vi "PBPCIcard_load.vi"(0 "PulseBlaster\nVLIW Array":T1(array[cluster])=[{"Output Bits"=16777215, "Data Field"=0, "OP Code"=0, "Delay Count"=20}, {"Output Bits"=0, "Data Field"=0, "OP Code"=3, "Delay Count"=20}, {"Output Bits"=0, "Data Field"=0, "OP Code"=6, "Delay Count"=60}] {"OP Code" format="%.0x"; "Output Bits" format="%.0x"}, 1 "Bytes/Word":u8=10, 2 "Memory":bool, 3 "error in (no error)":errorcluster, 4 "Base Address":u32 format="%.0x") -> (7 "error out":errorcluster)   [LabVIEW 2013]
doc: "PBcard_load: \nThis vi \n1) resets the PB, (consists of 4 steps)\n2) writes an array of VLIW's (very long instruction word) to the PB memory\n3) sends \"program finished\".\nAfter completion, a \"start\" command to the PB will make it run the programmed sequence. \n\nThe VLIW is implemented as a cluster of four integers (24bit, 20bit, 4bit, 32bit).\n\nNOTE: NO ERROR CHECKING IS PERFORMED. Error checking is supposedly taken care of before the VLIW array image is made, for example by Add_VLIW, which writes a PulseBlaster command to an array in memory. An"
uses:
  pbcomm8.vi
  pbcomm16.vi
  pbcomm32.vi
panel:
  # "External"
  # "Internal"
  # "(24 bits)"
  # "(20 bits)"
  # "(4 bits)"
  # "(32 bits)"
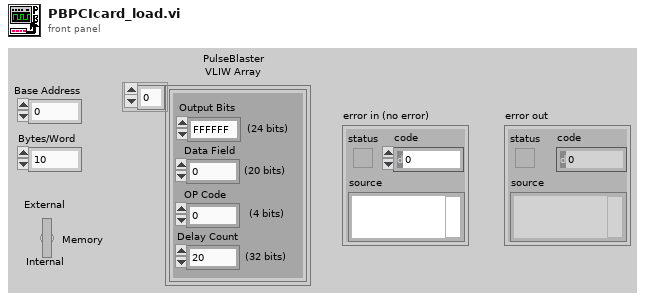
[diagram p1: front panel]
types:
  T1 = cluster{"Output Bits":u32, "Data Field":u32, "OP Code":u8, "Delay Count":u32}[]
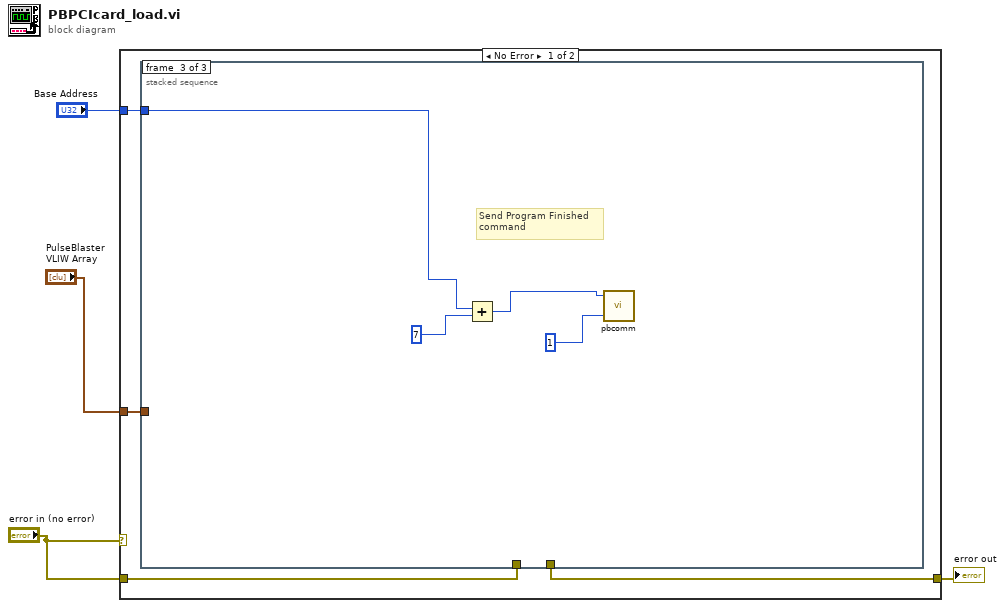
[diagram p0: block diagram]
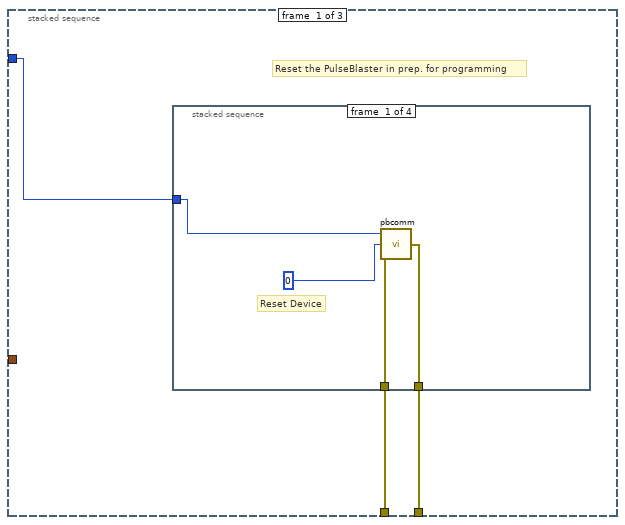
[diagram p2: hidden frame]
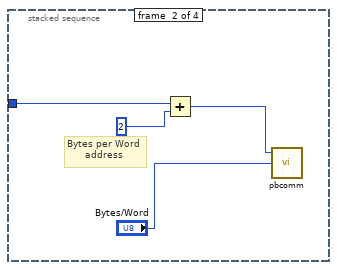
[diagram p3: hidden frame]
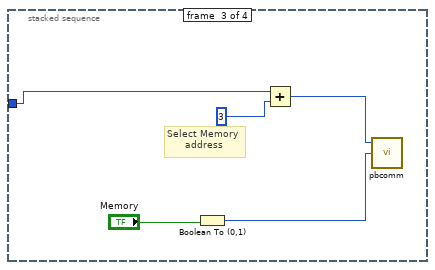
[diagram p4: hidden frame]
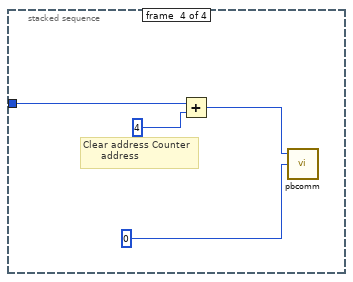
[diagram p5: hidden frame]
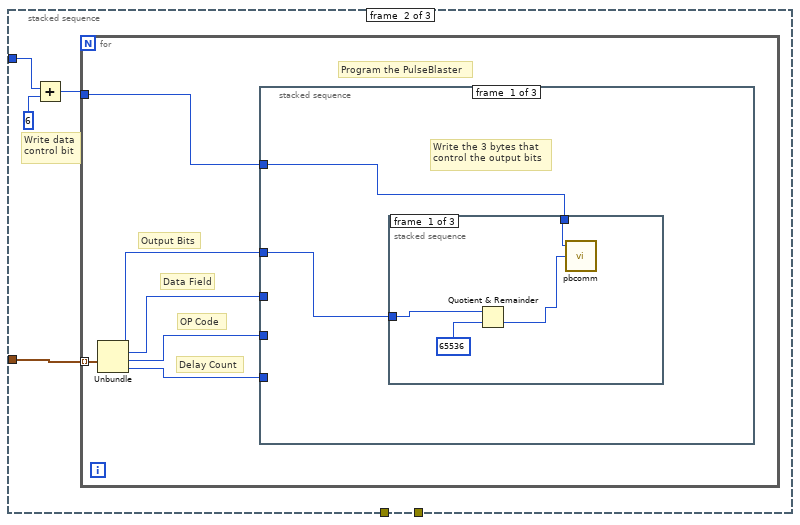
[diagram p6: hidden frame]
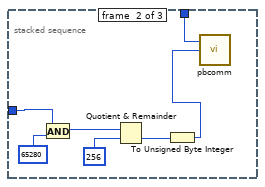
[diagram p7: hidden frame]
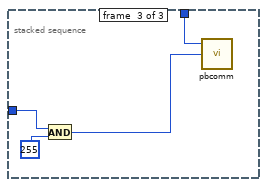
[diagram p8: hidden frame]
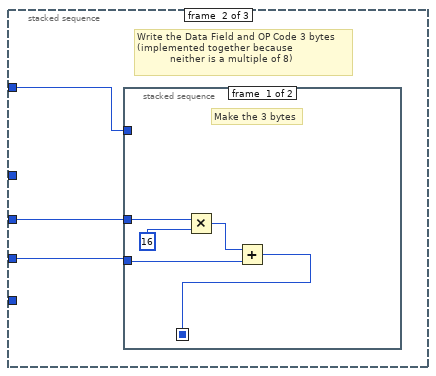
[diagram p9: hidden frame]
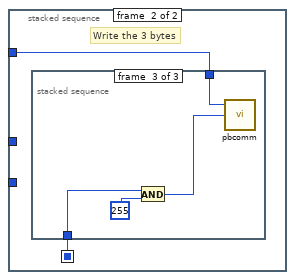
[diagram p10: hidden frame]
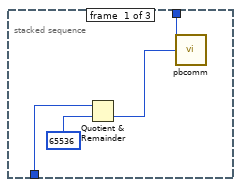
[diagram p11: hidden frame]
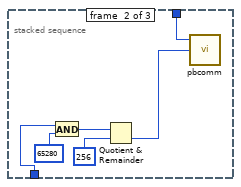
[diagram p12: hidden frame]
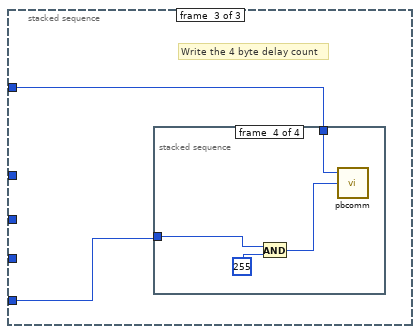
[diagram p13: hidden frame]
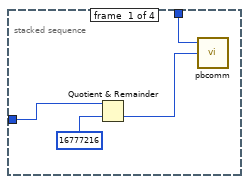
[diagram p14: hidden frame]
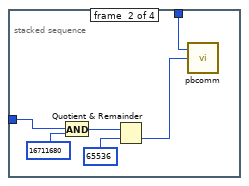
[diagram p15: hidden frame]
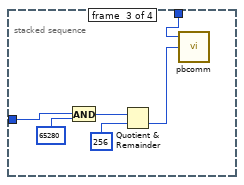
[diagram p16: hidden frame]
diagram:
  n1 = case shown="No Error" "error in (no error)" {
    tunnel: "PulseBlaster\nVLIW Array" -> [w8 _]
    tunnel: "Base Address" -> [w7 _]
    tunnel: "error in (no error)" -> [w6 w106]
    tunnel: [w5 w106] -> w1
    frame No Error {
      n2 = stacked-sequence {
        tunnel: w8 -> [_ w29 _]
        tunnel: w7 -> [w11 w31 w102]
        tunnel: w6 -> [w10 _ _]
        tunnel: [w9 _ _] -> w5
        frame #0 {
          # "Reset the PulseBlaster in prep. for programming"
          n3 = stacked-sequence {
            tunnel: w11 -> [w15 w19 w21 w25]
            tunnel: w10 -> [w13 _ _ _]
            tunnel: [w12 _ _ _] -> w9
            frame #0 {
              # "Reset Device"
              n4 = call-poly "pbcomm.vi"("error in"=w13, "write value"=u8 0, "address"=w15) -> ("error out"=w12:errorcluster)
            }
            frame #1 {
              # "Bytes per Word\n      address"
              n5 = Add(x=w19, y=u8 2) -> (x+y=w17:u32)
              n6 = call-poly "pbcomm.vi"("write value"="Bytes/Word", "address"=w17) -> ()  [unwired: 1 in, 1 out]
            }
            frame #2 {
              # "Select Memory\n      address"
              n7 = Boolean To (0,1)(Boolean="Memory") -> (0, 1=w20:i16)
              n8 = Add(x=w21, y=u8 3) -> (x+y=w23:u32)
              n9 = call-poly "pbcomm.vi"("write value"=w20, "address"=w23) -> ()  [unwired: 1 in, 1 out]
            }
            frame #3 {
              # "Clear address Counter\n      address"
              n10 = Add(x=w25, y=u8 4) -> (x+y=w27:u32)
              n11 = call-poly "pbcomm.vi"("write value"=u8 0, "address"=w27) -> ()  [unwired: 1 in, 1 out]
            }
          }
        }
        frame #1 {
          # "Write data\ncontrol bit"
          n12 = Add(x=w31, y=6) -> (x+y=w30:u32)
          n13 = for {
            tunnel: w30 -> [w38]
            tunnel: w29 -> [w33] mode=indexing
            # "Program the PulseBlaster"
            # "Delay Count"
            # "OP Code"
            # "Data Field"
            # "Output Bits"
            n14 = Unbundle(w33) -> ("Output Bits"=w37:u32, "Data Field"=w36:u32, "OP Code"=w35:u8, "Delay Count"=w34:u32)
            n15 = stacked-sequence {
              tunnel: w37 -> [w40 _ _]
              tunnel: w36 -> [_ w58 _]
              tunnel: w35 -> [_ w57 _]
              tunnel: w38 -> [w39 w56 w80]
              tunnel: w34 -> [_ _ w81]
              frame #0 {
                # "Write the 3 bytes that \ncontrol the output bits"
                n16 = stacked-sequence {
                  tunnel: w40 -> [w43 w49 w54]
                  tunnel: w39 -> [w42 w47 w52]
                  frame #0 {
                    n17 = Quotient & Remainder(x=w43, y=u32 65536) -> (floor(x/y)=w41:u32)  [unwired: 1 out]
                    n18 = call-poly "pbcomm.vi"("write value"=w41, "address"=w42) -> ()  [unwired: 1 in, 1 out]
                  }
                  frame #1 {
                    n19 = And(x=w49, y=u32 65280) -> (x .and. y?=w48:u32)
                    n20 = Quotient & Remainder(x=w48, y=u32 256) -> (floor(x/y)=w46:u32)  [unwired: 1 out]
                    n21 = To Unsigned Byte Integer(number=w46) -> (unsigned 8bit integer=w45:u8)
                    n22 = call-poly "pbcomm.vi"("write value"=w45, "address"=w47) -> ()  [unwired: 1 in, 1 out]
                  }
                  frame #2 {
                    n23 = And(x=w54, y=u32 255) -> (x .and. y?=w53:u32)
                    n24 = call-poly "pbcomm.vi"("write value"=w53, "address"=w52) -> ()  [unwired: 1 in, 1 out]
                  }
                }
              }
              frame #1 {
                # "Write the Data Field and OP Code 3 bytes\n(implemented together because \n           neither is a multiple of 8)"
                n25 = stacked-sequence {
                  seq-local: [w59 _] -> [_ w65]
                  tunnel: w58 -> [w61 _]
                  tunnel: w57 -> [w62 _]
                  tunnel: w56 -> [_ w64]
                  frame #0 {
                    # "Make the 3 bytes"
                    n26 = Multiply(x=w61, y=u32 16) -> (x*y=w60:u32)
                    n27 = Add(x=w60, y=w62) -> (x+y=w59:u32)
                  }
                  frame #1 {
                    # "Write the 3 bytes"
                    n28 = stacked-sequence {
                      tunnel: w65 -> [w67 w71 w77]
                      tunnel: w64 -> [w66 w70 w76]
                      frame #0 {
                        n29 = Quotient & Remainder(x=w67, y=u32 65536) -> (floor(x/y)=w68:u32)  [unwired: 1 out]
                        n30 = call-poly "pbcomm.vi"("write value"=w68, "address"=w66) -> ()  [unwired: 1 in, 1 out]
                      }
                      frame #1 {
                        n31 = And(x=w71, y=u32 65280) -> (x .and. y?=w73:u32)
                        n32 = Quotient & Remainder(x=w73, y=u32 256) -> (floor(x/y)=w72:u32)  [unwired: 1 out]
                        n33 = call-poly "pbcomm.vi"("write value"=w72, "address"=w70) -> ()  [unwired: 1 in, 1 out]
                      }
                      frame #2 {
                        n34 = And(x=w77, y=u32 255) -> (x .and. y?=w78:u32)
                        n35 = call-poly "pbcomm.vi"("write value"=w78, "address"=w76) -> ()  [unwired: 1 in, 1 out]
                      }
                    }
                  }
                }
              }
              frame #2 {
                # "Write the 4 byte delay count"
                n36 = stacked-sequence {
                  tunnel: w81 -> [w84 w88 w94 w100]
                  tunnel: w80 -> [w82 w87 w93 w98]
                  frame #0 {
                    n37 = Quotient & Remainder(x=w84, y=u32 16777216) -> (floor(x/y)=w83:u32)  [unwired: 1 out]
                    n38 = call-poly "pbcomm.vi"("write value"=w83, "address"=w82) -> ()  [unwired: 1 in, 1 out]
                  }
                  frame #1 {
                    n39 = And(x=w88, y=u32 16711680) -> (x .and. y?=w89:u32)
                    n40 = Quotient & Remainder(x=w89, y=u32 65536) -> (floor(x/y)=w86:u32)  [unwired: 1 out]
                    n41 = call-poly "pbcomm.vi"("write value"=w86, "address"=w87) -> ()  [unwired: 1 in, 1 out]
                  }
                  frame #2 {
                    n42 = And(x=w94, y=u32 65280) -> (x .and. y?=w95:u32)
                    n43 = Quotient & Remainder(x=w95, y=u32 256) -> (floor(x/y)=w92:u32)  [unwired: 1 out]
                    n44 = call-poly "pbcomm.vi"("write value"=w92, "address"=w93) -> ()  [unwired: 1 in, 1 out]
                  }
                  frame #3 {
                    n45 = And(x=w100, y=u32 255) -> (x .and. y?=w99:u32)
                    n46 = call-poly "pbcomm.vi"("write value"=w99, "address"=w98) -> ()  [unwired: 1 in, 1 out]
                  }
                }
              }
            }
          }
        }
        frame #2 {
          # "Send Program Finished \ncommand"
          n47 = Add(x=w102, y=7) -> (x+y=w104:u32)
          n48 = call-poly "pbcomm.vi"("write value"=1, "address"=w104) -> ()  [unwired: 1 in, 1 out]
        }
      }
    }
    frame Error {
    }
  }
  "error out" <- w1
